vi "Event Nested.vi"(8 "Alias":string, 10 "Msg":refnum<class "Msg.lvclass">, 11 "jettl Queue Actor in":refnum<class "jettl Queue Actor.lvclass">) -> (3 "jettl Queue Actor out":refnum<class "jettl Queue Actor.lvclass">)   [LabVIEW 2021, in "jettl.lvlib" / "jettl Queue Actor.lvlib" / "jettl Queue Actor.lvclass"]
uses:
  jettl Queue Actor.lvclass
  Actor/Msg/Msg.lvclass
  jettl Queue Actor.lvclass/jettl Queue Actor.ctl
  jettl.lvlib
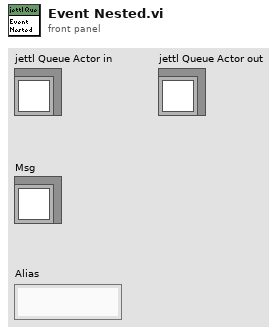
[diagram p1: front panel]
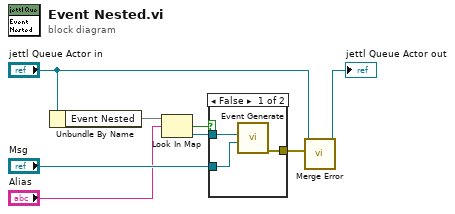
[diagram p0: block diagram]
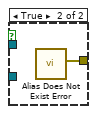
[diagram p2: hidden frame]
diagram:
  n1 = Unbundle By Name("jettl Queue Actor in") -> ("Event Nested"=w7:map{string, refnum<data-value>})
  n2 = Look In Map(map=w7, key="Alias") -> (key not found?=w6:bool, value=w8:refnum<data-value>)  [unwired: 1 in]
  n3 = case shown="False" w6 {
    tunnel: [w9 w12] -> w5
    tunnel: "Msg" -> [w10 _]
    tunnel: w8 -> [w11 _]
    frame False {
      n4 = call "Event Generate.vi"("Msg"=w10, "Event"=w11) -> ("error out"=w9:errorcluster)  [unwired: 9 in]
    }
    frame True {
      n5 = call "Alias Does Not Exist Error.vi"() -> ("Error"=w12:errorcluster)  [unwired: 11 in]
    }
  }
  n6 = call-dynamic "Merge Error.vi"("Error"=w5, "jettl Queue Actor in"="jettl Queue Actor in") -> ("jettl Queue Actor out"=→"jettl Queue Actor out":refnum<class "jettl Queue Actor.lvclass">)  [unwired: 9 in]
